vi "Async Get image from CamServer.vi"(1 "Image name":string="test", 2 "Image directory path":path=path "C:/test", 3 "Camera":T1="Travcam") -> (0 "Error out":errorcluster)   [LabVIEW 2015]
doc: "Asynchronously gets a snapshot image from the selected camera on the camera server and saves it to the specified path with specified name."
uses:
  Camera enum/Camera enum.ctl
  Globals/CamServer global.vi
panel:
  # "PN 21/08/15"
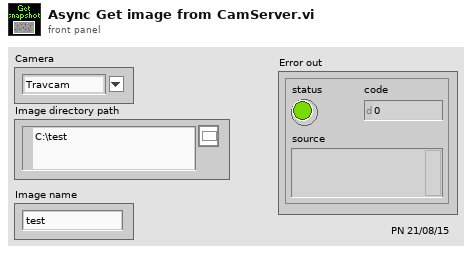
[diagram p1: front panel]
types:
  T1 = typedef "Camera enum.ctl" = string
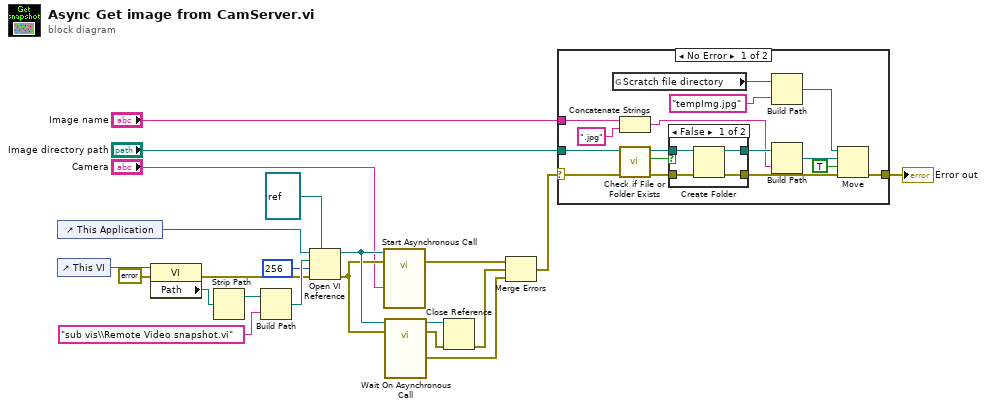
[diagram p0: block diagram]
diagram:
  n1 = control-ref of="This Application"() -> (w17:refnum<vi>)
  n2 = control-ref of="This VI"() -> (w22:refnum<vi>)
  n3 = property class="VI"(reference=w22, error in=errorcluster {"status"=FALSE, "code"=0, "source"=""} ("error in (no error)")) -> (error out=w19:errorcluster, "Path"=w15:path)  [unwired: 1 out]
  n4 = Strip Path(path=w15) -> (stripped path=w14:path)  [unwired: 1 out]
  n5 = Build Path(base path=w14, name or relative path="sub vis\\Remote Video snapshot.vi") -> (appended path=w20:path)
  n6 = Open VI Reference(type specifier VI Refnum (for type only)=refnum<vi> refnum, application reference (local)=w17, vi path=w20, options=256, error in (no error)=w19) -> (vi reference=w13:refnum<vi>, error out=w12:errorcluster)  [unwired: 1 in]
  n7 = call-by-ref "Start Asynchronous Call"(reference=w13, error in=w12, "Camera"="Camera") -> (error out=w10:errorcluster)  [unwired: 2 out]
  n8 = call-by-ref "Wait On Asynchronous Call"(reference=w13, error in=w12) -> (reference out=w11:refnum<vi>, error out=w9:errorcluster, "Error out"=w7:errorcluster)  [unwired: 1 in]
  n9 = Close Reference(reference=w11, error in (no error)=w9) -> (error out=w8:errorcluster)
  n10 = Merge Errors(w10, w8, w7) -> (w4:errorcluster)
  n11 = case shown="No Error" w4 {
    selector: w4 -> [w37 w45]
    tunnel: "Image directory path" -> [w38 _]
    tunnel: "Image name" -> [w30 _]
    tunnel: [w28 w45] -> w1
    frame No Error {
      n12 = global read "CamServer global.vi" "Scratch file directory"() -> (w24:path)
      n13 = Concatenate Strings(w30, ".jpg" ("string")) -> (w27:string)
      n14 = call <vilib>:"Check if File or Folder Exists.vi"("error in (no error)"=w37, "path"=w38) -> ("error out"=w34:errorcluster, "file or folder exists?"=w36:bool, "dup path"=w35:path)  [unwired: 7 in]
      n15 = case shown="False" w36 {
        tunnel: w35 -> [w42 w44]
        tunnel: w34 -> [w41 w43]
        tunnel: [w40 w44] -> w31
        tunnel: [w39 w43] -> w32
        frame False {
          n16 = Create Folder(path (use dialog)=w42, error in=w41) -> (created path=w40:path, error out=w39:errorcluster)  [unwired: 1 in, 1 out]
        }
        frame True {
        }
      }
      n17 = Build Path(base path=w24, name or relative path="tempImg.jpg") -> (appended path=w23:path)
      n18 = Build Path(base path=w31, name or relative path=w27) -> (appended path=w29:path)
      n19 = Move(source path=w23, error in=w32, 9:TRUE ("overwrite (F)"), 10:w29) -> (error out=w28:errorcluster)  [unwired: 1 in, 2 out]
    }
    frame Error {
    }
  }
  "Error out" <- w1
